vi "HEWH RLT PRAT.vi"() -> ()   [LabVIEW 2023] (continued)
      n65 = call "HEWH GEA Notifier.vi"("Status"=UTILITY_Notifier."Set", "error in (no error)"=w173, "name (unnamed)"="GEA_B") -> ("error out"=w172:errorcluster)  [unwired: 7 in, 1 out]
      n66 = call "HEWH GEA Notifier.vi"("Status"=UTILITY_Notifier."Set", "error in (no error)"=w172, "name (unnamed)"="GEA_C") -> ("error out"=w171:errorcluster)  [unwired: 7 in, 1 out]
      n67 = call "HEWH GEA Notifier.vi"("Status"=UTILITY_Notifier."Set", "error in (no error)"=w171, "name (unnamed)"="GEA_D") -> ("error out"=w141:errorcluster)  [unwired: 7 in, 1 out]
      n68 = Bundle By Name(cluster="File Locations In", "General Setup Paths.Tool Base Path"=w188) -> (w191:T3)
      n69 = call "UTILITY String Notifier.vi"("Status"=UTILITY_Notifier."Set", "error in (no error)"=w141, "Set Status"="", "name (unnamed)"="GasThermalEff") -> ("error out"=w140:errorcluster)  [unwired: 6 in, 1 out]
      n70 = call "HEWH Gas Notifier.vi"("Status"=UTILITY_Notifier."Set", "error in (no error)"=w140, "name (unnamed)"="GasData") -> ("error out"=w134:errorcluster)  [unwired: 7 in, 1 out]
      n71 = case shown="\"Four Stations\"" w187 {
        tunnel: [w251 w265] -> w185
        tunnel: [w251 w264] -> w184
        tunnel: [w251 w263] -> w183
        tunnel: [w249 w262] -> w108
        tunnel: [w249 w261] -> w107
        tunnel: [w249 w260] -> w106
        tunnel: w191 -> [_ w256]
        tunnel: [w250 w259] -> w167
        tunnel: [w250 w258] -> w166
        tunnel: [w250 w257] -> w165
        tunnel: errorcluster {"status"=FALSE, "code"=0, "source"=""} ("error out") -> [w248 w252]
        tunnel: [w248 w253] -> w129
        frame "Single Station", Default {
          w249 = refnum<k24> refnum (".NET Refnum in")
          w250 = T3 {"General Setup Paths"={"Calibration File Path"=path "", "DOE Capacity Path"=path "", "Data Folder Path"=path "", "RLT Backup Data Path"=path "", "Tool Base Path"=path "", "General Startup Config Path"=path "", "File Save Previous Run Path"=path "", "File Save Configuration Data Path"=path ""}, "Data File Paths"={"Data File Path"=path "", "Debug File Path"=path "", "Bus Log Path"=path "", "Current"=path "", "Summary"=path ""}, "New Summary Created"=FALSE, "Check Location Interval (Second)"=0} ("File Locations Out")
          w251 = T31 {"Appliance Details"={"FileVersionInfo"={"FileVersion"="", "ProductName"="", "InternalName"="", "CompanyName"="", "LegalCopyright"="", "FileDescription"=""}, "Dishwasher Info"={"Open Cup Weight (gm):"=0.0, "Auto Cup Weight (gm):"=0.0, "Detergent-Dish:"="", "Inlet Temperature-Dish:"="", "Cycle Mode-Dish:"="", "Unit Control-Dish:"="", "Manufacturer-Dish:"=""}, "Washer Info"={"Hot Water Temperature (Fahrenheit):"="", "Cold Water Temperature (Fahrenheit):"="", "Capacity (cu.ft):"=0.0, "Initial Cloth Weight:"=0.0, "Cloth Lot:"=0, "Model Family:"="", "Program Name:"="", "Cycle Selection:"="", "Wash Temperature:"="", "Rinse Temperature:"="", "Load Size:"=""}, "File Name Output Array"=[], "Calibration Output Array"=[], "Appliance Common"={"Engineer:"="", "Model Number:"="", "Serial Number:"="", "Comments:"="", "Station ID:"="", "Technician:"="", "TR Number:"="", "Lab ID:"="", "Voltage:"="", "Water Pressure (PSI):"="", "Test Date:"="", "Computer Name:"="", "IP Address:"="", "Ambient RH:"="", "Frequency:"="", "Build:"="", "Filename:"="", "Test Type:"="", "Load Run #:"=0, "Ambient Temperature (F):"="", "File Path:"=path "", "Cycles Per Year"=60}, "Water Heater"={"Heating Mode:"=""}, "Dryer"={"Heat Setting:"="", "Washer Water Temperature (60 ± 5°F):"=60, "Water Hardness (PPM):"=17, "Dryness Setting:"="", "Dryer Type:"="", "Exhaust:"="", "Drying Cycle:"="", "Load Type:"="", "Nominal Load Weight"="", "Dryer Initial IMC Data"={"Measured IMC (lbs)"=7.0, "Actual Initial RMC (%)"=7.0, "RMC (Desired %)"=100.0, "Bone Dry Wt(lbs)"=7.0, "Tolerance(%)"=5.0, "Actual Final RMC (%)"=0.0, "CEF (lbf/kWh)"=0.0, "Minimum Weight (lbf)"=0.0, "Average Weight (lbf)"=0.0, "Maximum Weight (lbf)"=0.0, "Measured IMC In Range?"=FALSE, "Moisture Reduction Factor"=55.5, "Field Use Factor"=1.04, "Empty Dryer Cold Weigth"=0.0, "Energy Standard"=enum."D2-Automatic Dryer", "Weight Cloth (lbs)"=0.0, "Relative Moisture Content (%)"=0.0, "Relative Moisture Content - Avg (%)"=0.0}}}, "Display Data (RLT)"={"Status Color"=0, "Serial Number Display"="", "Cycle Count Display"=0, "Station Label Display"="", "Current Run Start Time Display"=0.0, "Board ID Display"="", "RPM Display"=0, "Current Display"=0.0, "Current Path Display"=path "", "Saving Display"=FALSE, "Unit Type Display"=enum."", "Total Time On Display"=0.0, "UI Button"=FALSE}} ("Main Washer Display Out")
          # "GEA Information Out"
        }
        frame "Four Stations" {
          n72 = call "UTILITY Read Config File Start BUS.vi"("Error In"=w252, "Station ID"="StationD", "File Locations In"=w256) -> ("Error Out"=w255:errorcluster, "Main Washer Display Out"=w263:T31, "GEA3 Reference Out"=w260:refnum<k24>, "File Locations Out"=w257:T3)  [unwired: 5 in]
          n73 = call "UTILITY Read Config File Start BUS.vi"("Error In"=w255, "Station ID"="StationC", "File Locations In"=w256) -> ("Error Out"=w254:errorcluster, "Main Washer Display Out"=w264:T31, "GEA3 Reference Out"=w261:refnum<k24>, "File Locations Out"=w258:T3)  [unwired: 5 in]
          n74 = call "UTILITY Read Config File Start BUS.vi"("Error In"=w254, "Station ID"="StationB", "File Locations In"=w256) -> ("Error Out"=w253:errorcluster, "Main Washer Display Out"=w265:T31, "GEA3 Reference Out"=w262:refnum<k24>, "File Locations Out"=w259:T3)  [unwired: 5 in]
        }
      }
      n75 = call "UTILITY Boolean Notifier.vi"("Status"=UTILITY_Notifier."Set", "error in (no error)"=w134, "Set Status"=FALSE, "name (unnamed)"="Splash") -> ("error out"=w121:errorcluster)  [unwired: 6 in, 1 out]
      n76 = call "HEWH MW100 Data.vi"("Status"=UTILITY_Notifier."Set", "error in (no error)"=w121, "name (unnamed)"="MW100") -> ("error out"=w120:errorcluster)  [unwired: 7 in, 1 out]
      n77 = call "HEWH Emerson Data.vi"("Status"=UTILITY_Notifier."Set", "error in (no error)"=w120, "name (unnamed)"="Emerson") -> ("error out"=w114:errorcluster)  [unwired: 7 in, 1 out]
      n78 = call "UTILITY String Notifier.vi"("Status"=UTILITY_Notifier."Set", "error in (no error)"=w114, "Set Status"="", "name (unnamed)"="Scan_Rate") -> ("error out"=w111:errorcluster)  [unwired: 6 in, 1 out]
      n79 = call "UTILITY Read Config File Start BUS.vi"("Error In"=w129, "Station ID"="StationA", "File Locations In"=w191) -> ("Main Washer Display Out"=w186:T31, "GEA3 Reference Out"=w109:refnum<k24>, "File Locations Out"=w168:T3)  [unwired: 5 in, 1 out]
      n80 = call "HEWH HHV Notifier.vi"("Status"=UTILITY_Notifier."Set", "error in (no error)"=w111, "name (unnamed)"="HHVData") -> ("error out"=w104:errorcluster)  [unwired: 7 in, 1 out]
      n81 = Obtain Notifier(name (unnamed)="SplashScreen", notification data type=FALSE ("Init Complete"), error in (no error)=w104) -> (notifier out=w130:refnum<notifier>, error out=w131:errorcluster)  [unwired: 1 in, 1 out]
    }
    frame Enabled {
    }
  }
  n82 = disable-structure shown="Disabled" {
    disable-tunnel: w100 -> [w289 _]
    disable-tunnel: w99 -> [w288 _]
    disable-tunnel: w96 -> [w286 _]
    disable-tunnel: w95 -> [w285 _]
    disable-tunnel: w57 -> [w284 _]
    frame Disabled {
      # "Do the stuff associated with a draw"
      n83 = while {
        tunnel: w284 -> [w290]
        tunnel: [w290] -> w287
        stop <- w291 stop-if-true
        # "Make sure you get correct info during start"
        n84 = local read "Start Draw Loop"() -> (w291:bool)
        n85 = Wait Until Next ms Multiple(millisecond multiple=u32 250) -> ()  [unwired: 1 out]
      }
      n86 = while {
        tunnel: w287 -> [w303]
        tunnel: [w312] -> _
        tunnel: w286 -> [w311]
        tunnel: w289 -> [w298]
        tunnel: w288 -> [w299]
        tunnel: w285 -> [w295]
        i -> [w310]
        stop <- w309 stop-if-true
        n87 = Dequeue Element(queue=w298, error in (no error)=w303) -> (element=w300:T81, error out=w302:errorcluster)  [unwired: 1 in, 2 out]
        n88 = local read "Finish"() -> (w309:bool)
        n89 = Unbundle By Name(w300) -> ("Start Draw"=w296:bool, "Station ID"=w301:T26, "Station Draw Info"=w297:T15, "Send Condition"=w294:T2, "Disable Purge Pressurization"=w293:bool)
        "Start Draw" <- w296
        n90 = Wait Until Next ms Multiple(millisecond multiple=u32 100) -> ()  [unwired: 1 out]
        n91 = case shown="\"A\", Default" w301 {
          tunnel: [w313 w314 w315 w316] -> w307
          frame "A", Default {
            n92 = local read "Disable Station 1"() -> (w313:T34)
          }
          frame "B" {
            n93 = local read "Disable Station 2"() -> (w314:T34)
          }
          frame "C" {
            n94 = local read "Disable Station 3"() -> (w315:T34)
          }
          frame "D" {
            n95 = local read "Disable Station 4"() -> (w316:T34)
          }
        }
        n96 = Equal?(x=HEWH_RLT_Station_Disable."Enable Station", y=w307) -> (x = y?=w305:bool)
        n97 = And(x=w296, y=w305) -> (x .and. y?=w304:bool)
        n98 = case shown="True" w304 {
          tunnel: w302 -> [w317 w347]
          tunnel: [w317 w321] -> w312
          tunnel: w311 -> [_ w343]
          tunnel: w301 -> [_ w339]
          tunnel: w299 -> [_ w323]
          tunnel: w297 -> [_ w335]
          tunnel: w295 -> [_ w324]
          tunnel: w294 -> [_ w338]
          tunnel: w293 -> [_ w334]
          frame False {
          }
          frame True {
            # "This is everything required to draw water"
            n99 = flat-sequence {
              tunnel: w347 -> [w457]
              tunnel: [w457] -> w333
              frame #0 {
                n100 = property on="Scan Rate (Seconds)" class="DigNum (strict)"("Value"=T11 30.0 ("Scan Rate (Seconds)")) -> ()  [unwired: 2 in, 2 out]
                n101 = local write "Draw Complete"(FALSE ("Draw Complete")) -> ()
              }
            }
            n102 = local read "Intellifaucet Open Greater 2.2 GPM"() -> (w326:dbl)
            n103 = local read "Intellifaucet Open Less  2.2 GPM"() -> (w327:dbl)
            n104 = local read "Intellifaucet Open Less 1_7 GPM"() -> (w328:dbl)
            n105 = local read "Intellifaucet Open Less 1 GPM"() -> (w329:dbl)
            n106 = local read "Ritter Gas Drum Meter"() -> (w318:bool)
            n107 = control-ref of="Scan Rate (Seconds)"() -> (w319:refnum<vi>)
            n108 = local read "K-Factor (Flow)"() -> (w337:dbl)
            n109 = local read "Test Fixture Hardware Draw Loop"() -> (w332:T55)
            n110 = local read "Intellifaucet Type"() -> (w336:string)
            n111 = local read "Pressurize Tank?"() -> (w341:bool)
            n112 = local read "K-Factor (Temperature)"() -> (w340:dbl)
            n113 = case shown="\"A\", Default" w339 {
              tunnel: w333 -> [w371 w394 w417 w440]
              tunnel: "Purge Time (Seconds)" -> [w370 w391 w414 w439]
              tunnel: [w361 w384 w407 w430] -> w346
              tunnel: w335 -> [w369 w390 w409 w438]
              tunnel: "Skip Purge" -> [w367 w392 w416 w437]
              tunnel: "Skip Draw" -> [w366 w393 w415 w436]
              tunnel: w343 -> [w368 w387 w412 w435]
              tunnel: w341 -> [w363 w386 w411 w432]
              tunnel: w340 -> [w362 w385 w410 w431]
              tunnel: w338 -> [w360 w383 w406 w429]
              tunnel: w337 -> [w359 w382 w405 w428]
              tunnel: w336 -> [w358 w381 w404 w427]
              tunnel: w334 -> [w357 w380 w403 w426]
              tunnel: w332 -> [w356 w379 w402 w425]
              tunnel: "Pressurization Time (sec)" -> [w355 w378 w401 w424]
              tunnel: "NOx Purge Time" -> [w354 w377 w400 w423]
              tunnel: w329 -> [w353 w376 w399 w422]
              tunnel: w328 -> [w352 w375 w398 w421]
              tunnel: w327 -> [w351 w374 w397 w420]
              tunnel: w326 -> [w350 w373 w396 w419]
              tunnel: w319 -> [w349 _ _ _]
              tunnel: w318 -> [w348 w372 w395 w418]
              frame "A", Default {
                n114 = local read "Core HEWH Data Input A"() -> (w365:T13)
                n115 = call "HEWH Purge Draw Sequence.vi"("Intellifaucet Open Less 1 GPM"=w353, "Purge Time (Seconds)"=w370, "Intellifaucet Open Less 1_7 GPM"=w352, "Station Draw Info"=w369, "Current Cond"=w360, "Intellifaucet Open Less  2.2 GPM"=w351, "Intellifaucet Open Greater 2.2 GPM"=w350, "Error In"=w371, "Skip Purge"=w367, "Core HEWH Data Input"=w365, "Scan Rate (Seconds)"=w349, "Disable Purge Pressurization"=w357, "Skip Draw"=w366, "MW100 Sema"=w368, "K-Factor (Intellifaucet)"=w362, "Pressurize Tank while Heating?"=w363, "Intellifaucet Type"=w358, "Ritter Gas Drum Meter"=w348, "Test Fixture Hardware"=w356, "NOx Purge Time"=w354, "K-Factor (Flow)"=w359, "Pressurization Time (sec)"=w355) -> ("Core HEWH Data out"=→"Station A Update":T13, "Error Out"=w361:errorcluster)  [unwired: 4 in]
              }
              frame "B" {
                n116 = local read "Core HEWH Data Input B"() -> (w389:T13)
                n117 = call "HEWH Purge Draw Sequence.vi"("Intellifaucet Open Less 1 GPM"=w376, "Purge Time (Seconds)"=w391, "Intellifaucet Open Less 1_7 GPM"=w375, "Station Draw Info"=w390, "Current Cond"=w383, "Intellifaucet Open Less  2.2 GPM"=w374, "Intellifaucet Open Greater 2.2 GPM"=w373, "Error In"=w394, "Skip Purge"=w392, "Core HEWH Data Input"=w389, "Disable Purge Pressurization"=w380, "Skip Draw"=w393, "MW100 Sema"=w387, "K-Factor (Intellifaucet)"=w385, "Pressurize Tank while Heating?"=w386, "Intellifaucet Type"=w381, "Ritter Gas Drum Meter"=w372, "Test Fixture Hardware"=w379, "NOx Purge Time"=w377, "K-Factor (Flow)"=w382, "Pressurization Time (sec)"=w378) -> ("Core HEWH Data out"=→"Station B Update":T13, "Error Out"=w384:errorcluster)  [unwired: 5 in]
              }
              frame "C" {
                n118 = local read "Core HEWH Data Input C"() -> (w408:T13)
                n119 = call "HEWH Purge Draw Sequence.vi"("Intellifaucet Open Less 1 GPM"=w399, "Purge Time (Seconds)"=w414, "Intellifaucet Open Less 1_7 GPM"=w398, "Station Draw Info"=w409, "Current Cond"=w406, "Intellifaucet Open Less  2.2 GPM"=w397, "Intellifaucet Open Greater 2.2 GPM"=w396, "Error In"=w417, "Skip Purge"=w416, "Core HEWH Data Input"=w408, "Disable Purge Pressurization"=w403, "Skip Draw"=w415, "MW100 Sema"=w412, "K-Factor (Intellifaucet)"=w410, "Pressurize Tank while Heating?"=w411, "Intellifaucet Type"=w404, "Ritter Gas Drum Meter"=w395, "Test Fixture Hardware"=w402, "NOx Purge Time"=w400, "K-Factor (Flow)"=w405, "Pressurization Time (sec)"=w401) -> ("Core HEWH Data out"=→"Station C Update":T13, "Error Out"=w407:errorcluster)  [unwired: 5 in]
              }
              frame "D" {
                n120 = local read "Core HEWH Data Input D"() -> (w434:T13)
                n121 = call "HEWH Purge Draw Sequence.vi"("Intellifaucet Open Less 1 GPM"=w422, "Purge Time (Seconds)"=w439, "Intellifaucet Open Less 1_7 GPM"=w421, "Station Draw Info"=w438, "Current Cond"=w429, "Intellifaucet Open Less  2.2 GPM"=w420, "Intellifaucet Open Greater 2.2 GPM"=w419, "Error In"=w440, "Skip Purge"=w437, "Core HEWH Data Input"=w434, "Disable Purge Pressurization"=w426, "Skip Draw"=w436, "MW100 Sema"=w435, "K-Factor (Intellifaucet)"=w431, "Pressurize Tank while Heating?"=w432, "Intellifaucet Type"=w427, "Ritter Gas Drum Meter"=w418, "Test Fixture Hardware"=w425, "NOx Purge Time"=w423, "K-Factor (Flow)"=w428, "Pressurization Time (sec)"=w424) -> ("Core HEWH Data out"=→"Station D Update":T13, "Error Out"=w430:errorcluster)  [unwired: 5 in]
              }
            }
            n122 = flat-sequence {
              tunnel: w346 -> [w444]
              tunnel: w324 -> [w443]
              tunnel: [w442] -> w322
              tunnel: [w449] -> w325
              tunnel: w323 -> [w448]
              tunnel: w322 -> [w447]
              tunnel: w325 -> [w451]
              tunnel: [w451] -> w320
              tunnel: [w454] -> w321
              tunnel: w320 -> [w454]
              frame #0 {
                # "Increment cycle"
                n123 = Generate User Event(priority (normal)=usereventprio."high priority", user event=w443, event data cluster=TRUE ("Draw Start"), error in=w444) -> (error out=w442:errorcluster)  [unwired: 1 out]
              }
              frame #1 {
                # "Update draw stats"
                n124 = Generate User Event(priority (normal)=usereventprio."normal priority", user event=w448, event data cluster=TRUE ("event data"), error in=w447) -> (error out=w449:errorcluster)  [unwired: 1 out]
              }
              frame #2 {
              }
              frame #3 {
                n125 = property on="Scan Rate (Seconds)" class="DigNum (strict)"("Value"="Scan Rate (Default)") -> ()  [unwired: 2 in, 2 out]
                "Draw Complete" <- TRUE ("Draw Complete")
              }
            }
          }
        }
        "Draw Loop" <- w310
      }
    }
    frame Enabled {
    }
  }
  n126 = flat-sequence {
    tunnel: w57 -> [w459]
    tunnel: [w459] -> w74
    frame #0 {
      n127 = while {
        stop <- TRUE stop-if-true
        n128 = disable-structure shown="Disabled" {
          frame Disabled {
            n129 = local read "DAQ Complete"() -> ()  [unwired: 1 out]
          }
          frame Enabled {
          }
        }
        n130 = Wait (ms)(milliseconds to wait=u32 250) -> ()  [unwired: 1 out]
      }
      n131 = local write "Enable Auto Control"(FALSE ("Enable Auto Control")) -> ()
    }
  }
  n132 = disable-structure shown="Disabled" {
    disable-tunnel: [w466 _] -> w81
    disable-tunnel: w57 -> [w462 _]
    frame Disabled {
      # "Display messages. I need to work on this. \n\nIt was lower priority."
      n133 = Obtain Queue(name (unnamed)="ScanRate", element data type=FALSE, error in (no error)=w462) -> (queue out=w466:refnum<queue>, error out=w465:errorcluster)  [unwired: 2 in, 1 out]
      n134 = while {
        tunnel: w466 -> [w475]
        tunnel: w465 -> [w474]
        tunnel: [w473] -> w464
        tunnel: [w472] -> w463
        i -> [w469]
        stop <- w476 stop-if-true
        n135 = local read "DAQ Finished"() -> (w476:bool)
        n136 = call "HEWH Scan Rate Loop Trigger.vi"("Scan Rate (Seconds)"="Scan Rate (Seconds)", "Loop Index Input"=w469) -> ("Loop Trigger"=w470:bool)  [unwired: 7 in, 2 out]
        n137 = Enqueue Element(queue=w475, element=w470, error in (no error)=w474) -> (queue out=w472:refnum<queue>, error out=w473:errorcluster)  [unwired: 1 in, 1 out]
      }
      n138 = while {
        i -> [w477]
        stop <- w496 stop-if-true
        w491 = UTILITY_Notifier."Read" ("Status")
        n139 = call "UTILITY String Notifier.vi"("Status"=w491, "name (unnamed)"="Message") -> ("error out"=w495:errorcluster, "latest notification"=w483:string)  [unwired: 8 in]
        "Message" <- w483
        n140 = local read "Disable Station 1"() -> (w481:T34)
        n141 = call "UTILITY String Notifier.vi"("Status"=w491, "error in (no error)"=w495, "name (unnamed)"="MessageA") -> ("error out"=w494:errorcluster, "latest notification"=w486:string)  [unwired: 7 in]
        n142 = case shown="\"Enable Station\"" w481 {
          tunnel: w486 -> [_ w514]
          tunnel: w483 -> [_ w512]
          frame "Disable Station (No Draw)", Default {
          }
          frame "Enable Station" {
            n143 = call "HEWH Message Filter.vi"("Main Display?"=TRUE, "Station Message"=w514, "Main Message"=w512) -> ("Combined Message"=→"Message A" →"Message A Detail":string)  [unwired: 7 in, 1 out]
          }
        }
        n144 = local read "Disable Station 2"() -> (w480:T34)
        n145 = call "UTILITY String Notifier.vi"("Status"=w491, "error in (no error)"=w494, "name (unnamed)"="MessageB") -> ("error out"=w493:errorcluster, "latest notification"=w485:string)  [unwired: 7 in]
        n146 = case shown="\"Disable Station (No Draw)\", Default" w480 {
          tunnel: w485 -> [_ w510]
          tunnel: w483 -> [_ w508]
          frame "Disable Station (No Draw)", Default {
          }
          frame "Enable Station" {
            n147 = call "HEWH Message Filter.vi"("Main Display?"=TRUE, "Station Message"=w510, "Main Message"=w508) -> ("Combined Message"=→"Message B" →"Message B Detail":string)  [unwired: 7 in, 1 out]
          }
        }
        n148 = local read "Disable Station 3"() -> (w479:T34)
        n149 = call "UTILITY String Notifier.vi"("Status"=w491, "error in (no error)"=w493, "name (unnamed)"="MessageC") -> ("error out"=w492:errorcluster, "latest notification"=w484:string)  [unwired: 7 in]
        n150 = case shown="\"Disable Station (No Draw)\", Default" w479 {
          tunnel: w484 -> [_ w506]
          tunnel: w483 -> [_ w504]
          frame "Disable Station (No Draw)", Default {
          }
          frame "Enable Station" {
            n151 = call "HEWH Message Filter.vi"("Main Display?"=TRUE, "Station Message"=w506, "Main Message"=w504) -> ("Combined Message"=→"Message C" →"Message C Detail":string)  [unwired: 7 in, 1 out]
          }
        }
        n152 = local read "Disable Station 4"() -> (w478:T34)
        n153 = call "UTILITY String Notifier.vi"("Status"=w491, "error in (no error)"=w492, "name (unnamed)"="MessageD") -> ("latest notification"=w482:string)  [unwired: 7 in, 1 out]
        n154 = case shown="\"Enable Station\"" w478 {
          tunnel: w483 -> [_ w502]
          tunnel: w482 -> [_ w501]
          frame "Disable Station (No Draw)", Default {
          }
          frame "Enable Station" {
            n155 = call "HEWH Message Filter.vi"("Main Display?"=TRUE, "Station Message"=w501, "Main Message"=w502) -> ("Combined Message"=→"Message D" →"Message D Detail":string)  [unwired: 7 in, 1 out]
          }
        }
        n156 = Wait Until Next ms Multiple(millisecond multiple=u32 1000) -> ()  [unwired: 1 out]
        n157 = local read "DAQ Finished"() -> (w496:bool)
        "GEA3 Read Message Loop" <- w477
      }
      n158 = Release Queue(queue=w463, error in (no error)=w464) -> ()  [unwired: 1 in, 3 out]
    }
    frame Enabled {
    }
  }
  n159 = disable-structure shown="Disabled" {
    disable-tunnel: w102 -> [w531 _]
    disable-tunnel: w98 -> [w529 _]
    disable-tunnel: w96 -> [w528 _]
    disable-tunnel: w94 -> [w527 _]
    disable-tunnel: w93 -> [w526 _]
    disable-tunnel: w92 -> [w525 _]
    disable-tunnel: w91 -> [w524 _]
    disable-tunnel: w90 -> [w523 _]
    disable-tunnel: w87 -> [w522 _]
    disable-tunnel: w86 -> [w521 _]
    disable-tunnel: w85 -> [w520 _]
    disable-tunnel: w84 -> [w519 _]
    disable-tunnel: w83 -> [w518 _]
    disable-tunnel: w82 -> [w517 _]
    disable-tunnel: w81 -> [w516 _]
    frame Disabled {
      # "Get data from system"
      n160 = while "Data Acquisition Steps" {
        shift-right: [w552] -> _
        shift-left: _ -> [w551]
        shift-right: [w555] -> w515
        shift-left: w518 -> [w550]
        shift-right: [w554] -> _
        shift-left: w531 -> [w556]
        tunnel: w528 -> [w549]
        tunnel: w529 -> [w548]
        shift-right: [w544] -> _
        shift-left: string[] [] -> [w547]
        tunnel: w527 -> [w543]
        tunnel: w526 -> [w542]
        tunnel: w525 -> [w541]
        tunnel: w524 -> [w540]
        tunnel: w523 -> [w539]
        tunnel: w522 -> [w538]
        tunnel: w521 -> [w537]
        tunnel: w520 -> [w536]
        tunnel: w519 -> [w535]
        tunnel: w517 -> [w534]
        tunnel: w516 -> [w533]
        i -> [w532]
        stop <- w553 stop-if-true
        # "Data Acquisition Steps"
        n161 = call <vilib>:"Parse State Queue__JKI_lib_State_Machine.vi"("State Queue"=w556, "Error In (no error)"=w550) -> ("Remaining States"=w558:string, "Current State"=w546:string, "Arguments"=w557:string)  [unwired: 11 in]
        "DAQ State" <- w546
        n162 = case shown="\"Get Gas Data\"" w546 {
          selector: w546 -> [_ w681 _ _ _ _ _ _ _ _ _ _ _ _ _ _ _ _ _ _ _ _ _ _ _ _ _ _ _ _ _ _ _ _ _ _ _ _ _ _ _ _ _ _ _ _ _]
          tunnel: w558 -> [w571 w684 w696 w704 w716 w745 w792 w814 w833 w840 w850 w887 w913 w929 w938 w942 w955 w1005 w1041 w1077 w1113 w1136 w1153 w1170 w1187 w1203 w1220 w1245 w1327 w1352 w1379 w1398 w1428 w1458 w1487 w1540 w1573 w1601 w1629 w1657 w1694 w1709 w1733 w1757 w1781 w1792 w1819]
          tunnel: w557 -> [_ _ _ _ _ _ _ _ _ _ _ _ _ _ _ _ _ _ _ _ _ _ _ _ _ _ _ _ _ _ _ _ _ _ _ _ _ _ _ _ _ _ _ _ _ _ _]
          tunnel: [w569 w686 errorcluster {"status"=FALSE, "code"=0, "source"=""} ("error out") w700 w714 w718 w784 w800 w825 w838 w848 w877 w910 w922 w930 w940 w943 w995 w1033 w1069 w1105 w1128 w1148 w1165 w1182 w1191 w1207 w1239 w1318 w1338 w1365 w1395 w1424 w1454 w1483 w1524 w1553 w1599 w1627 w1655 w1692 w1700 w1724 w1748 w1772 w1793 w1805] -> w555
          tunnel: w550 -> [w564 w685 w692 w701 w714 w718 w775 w798 w823 w838 w848 w885 w911 w923 w934 w940 w943 w997 w1035 w1071 w1107 _ w1140 w1157 w1176 w1191 w1206 w1243 w1308 w1338 w1366 w1396 w1425 w1455 w1484 w1533 w1553 w1599 w1627 w1655 w1692 w1696 w1720 w1744 w1769 w1793 w1817]
          tunnel: [w570 w683 w695 w703 w715 w744 w791 w813 w832 w839 w849 w886 w912 w928 w937 w941 w954 w1004 w1040 w1076 w1112 w1137 w1154 w1171 w1188 w1202 w1219 w1244 w1326 w1351 w1378 w1397 w1427 w1457 w1486 w1539 w1572 w1600 w1628 w1656 w1693 w1708 w1732 w1756 w1780 w1792 w1819] -> w554
          tunnel: [_ _ _ w698 _ _ _ _ _ _ _ _ _ _ _ _ _ _ _ _ _ _ _ _ _ _ _ _ _ _ _ _ _ _ _ _ _ _ _ _ _ _ _ _ _ _ _] -> w553
          tunnel: [w568 w680 w691 w702 w713 w729 w790 w812 w831 w837 w844 w880 w905 w927 w936 w939 w953 w1003 w1039 w1075 w1111 w1135 w1152 w1169 w1186 w1201 w1218 w1236 w1325 w1350 w1377 w1394 w1423 w1453 w1482 w1538 w1567 w1592 w1618 w1648 w1691 w1702 w1725 w1749 w1773 w1791 w1798] -> w552
          tunnel: w551 -> [w567 w680 w691 w702 w713 _ w781 w812 w831 w837 w845 w882 w905 w927 w936 w939 w950 w1000 w1038 w1074 w1110 w1129 w1151 w1168 w1185 w1196 w1213 w1238 w1304 w1345 w1372 w1392 w1426 w1456 w1485 w1538 w1568 w1593 w1619 w1649 w1690 w1703 w1726 w1750 w1774 w1791 w1799]
          tunnel: w549 -> [_ _ _ _ _ _ w771 w802 w827 _ _ _ _ _ w933 _ _ w996 w1034 w1070 w1106 _ _ _ _ _ _ _ _ _ _ _ _ _ _ _ _ _ _ _ _ _ _ _ _ _ _]
          tunnel: w548 -> [w566 _ _ _ _ _ _ _ _ _ _ _ _ _ _ _ _ _ _ _ _ _ _ _ _ _ _ _ _ _ _ _ _ _ _ _ _ _ _ _ _ _ _ _ _ _ _]
          tunnel: w543 -> [_ _ _ _ _ _ _ _ _ _ _ _ _ _ _ _ w949 _ _ _ _ _ _ _ _ _ _ _ _ _ _ _ _ _ _ _ _ _ _ _ _ _ _ _ _ _ _]
          tunnel: w542 -> [_ _ _ _ _ _ _ _ _ _ _ _ _ _ _ _ _ _ _ _ _ _ _ _ _ _ _ _ _ _ _ w1391 _ _ _ _ _ _ _ _ _ _ _ _ _ _ _]
          tunnel: w541 -> [_ _ _ _ _ _ _ _ _ _ _ _ _ _ _ _ _ _ _ _ _ _ _ _ _ _ _ _ _ _ _ _ w1421 _ _ _ _ _ _ _ _ _ _ _ _ _ _]
          tunnel: w540 -> [_ _ _ _ _ _ _ _ _ _ _ _ _ _ _ _ _ _ _ _ _ _ _ _ _ _ _ _ _ _ _ _ _ w1451 _ _ _ _ _ _ _ _ _ _ _ _ _]
          tunnel: w539 -> [_ _ _ _ _ _ _ _ _ _ _ _ _ _ _ _ _ _ _ _ _ _ _ _ _ _ _ _ _ _ _ _ _ _ w1480 _ _ _ _ _ _ _ _ _ _ _ _]
          tunnel: w538 -> [_ _ _ _ _ _ _ _ _ _ w843 _ _ _ _ _ _ _ _ _ _ _ _ _ _ _ _ _ _ _ _ _ _ _ _ _ _ _ _ _ _ _ _ _ _ _ _]
          tunnel: w537 -> [_ _ _ _ _ _ _ _ _ _ w847 _ _ _ _ _ _ _ _ _ _ _ _ _ _ _ _ _ _ _ _ _ _ _ _ _ _ _ _ _ _ _ _ _ _ _ _]
          tunnel: w536 -> [_ _ _ _ _ _ _ _ _ _ w842 _ _ _ _ _ _ _ _ _ _ _ _ _ _ _ _ _ _ _ _ _ _ _ _ _ _ _ _ _ _ _ _ _ _ _ _]
          tunnel: w535 -> [_ _ _ _ _ _ _ _ _ _ w841 _ _ _ _ _ _ _ _ _ _ _ _ _ _ _ _ _ _ _ _ _ _ _ _ _ _ _ _ _ _ _ _ _ _ _ _]
          tunnel: w534 -> [_ _ _ _ _ _ w777 _ _ _ _ _ _ _ _ _ _ _ _ _ _ _ _ _ _ _ _ _ _ _ _ _ _ _ _ _ _ _ _ _ _ _ _ _ _ _ _]
          tunnel: w533 -> [w563 _ _ _ _ _ _ _ _ _ _ _ _ _ _ _ _ _ _ _ _ _ _ _ _ _ _ _ _ _ _ _ _ _ _ _ _ _ _ _ _ _ _ _ _ _ _]
          frame "", "Idle" {
            n163 = event shown="[0] Timeout" {
              selector: w566 -> [_ _ _ _]
              dyn-events: _ -> [_ _ _ _]
              timeout: "DAQ Timeout" -> [_ _ _ _]
              tunnel: w571 -> [w584 w599 w613 w614]
              tunnel: [w574 w600 w613 w615] -> w570
              tunnel: w567 -> [w582 w601 w607 w617]
              tunnel: [w578 w597 w612 w618] -> w569
              tunnel: w564 -> [w577 w597 w612 w619]
              tunnel: [w582 w601 w606 w622] -> w568
              tunnel: w563 -> [w576 _ _ _]
              event Timeout {
                # "Trigger data save"
                n164 = event-data() -> ()  [unwired: 1 in, 1 out]
                n165 = Unbundle By Name(w582) -> ("Core HEWH Data Input A.LV Program"=w581:T25)
                n166 = Dequeue Element(queue=w576, error in (no error)=w577) -> (element=w579:bool, error out=w578:errorcluster)  [unwired: 1 in, 2 out]
                n167 = case shown="True" w579 {
                  tunnel: ["" w596] -> w573
                  tunnel: w581 -> [_ w595]
                  frame False {
                  }
                  frame True {
                    n168 = local read "Final Headers B"() -> (w588:bool)
                    n169 = local read "Log Data Output (D)"() -> (w591:bool)
                    n170 = local read "Final Headers A"() -> (w589:bool)
                    n171 = local read "Final Headers C"() -> (w587:bool)
                    n172 = local read "Final Headers D"() -> (w586:bool)
                    n173 = local read "Log Data Output (C)"() -> (w592:bool)
                    n174 = local read "Log Data Output (A)"() -> (w594:bool)
                    n175 = local read "Log Data Output (B)"() -> (w593:bool)
                    n176 = call "HEWH Create Save Data States.vi"("LV Program"=w595, "Data Loop?"=TRUE, "Final Headers A"=w589, "Final Headers C"=w587, "Log Data Output (C)"=w592, "Log Data Output (A)"=w594, "Log Data Output (D)"=w591, "Log Data Output (B)"=w593, "Final Headers B"=w588, "Final Headers D"=w586) -> ("SM States"=w596:string)  [unwired: 8 in, 1 out]
                  }
                }
                n177 = call "HEWH Build States.vi"("LV Program"=w581) -> ("SM States"=w583:string, "Get Gas Data"=w580:bool, "Vesta Connect"=w572:bool)  [unwired: 12 in]
                n178 = call <vilib>:"Add State(s) to Queue__jki_lib_state_machine.vi"("State(s) in Front (\"\")"=w583, "State(s) in (\"\")"=w584) -> ("States Out"=w575:string)  [unwired: 13 in]
                n179 = call <vilib>:"Add State(s) to Queue__jki_lib_state_machine.vi"("State(s) in Front (\"\")"=w573, "State(s) in (\"\")"=w575) -> ("States Out"=w574:string)  [unwired: 13 in]
              }
              event "Finish": Value Change {
                n180 = event-data() -> ()  [unwired: 1 in, 6 out]
                n181 = call <vilib>:"Add State(s) to Queue__jki_lib_state_machine.vi"("State(s) in Front (\"\")"="Shutdown Equipment\nExit", "State(s) in (\"\")"=w599) -> ("States Out"=w600:string)  [unwired: 13 in]
              }
              event User Event {
                n182 = event-data() -> ()  [unwired: 1 in, 5 out]
                n183 = local read "Station A Update"() -> (w608:T13)
                n184 = local read "Station B Update"() -> (w609:T13)
                n185 = local read "Station C Update"() -> (w610:T13)
                n186 = local read "Station D Update"() -> (w611:T13)
                n187 = Unbundle By Name(w608) -> ("Calc and Calibration"=w605:T24)
                n188 = Unbundle By Name(w609) -> ("Calc and Calibration"=w604:T24)
                n189 = Unbundle By Name(w610) -> ("Calc and Calibration"=w603:T24)
                n190 = Unbundle By Name(w611) -> ("Calc and Calibration"=w602:T24)
                n191 = Bundle By Name(cluster=w607, "Core HEWH Data Input A.Calc and Calibration"=w605, "Core HEWH Data Input B.Calc and Calibration"=w604, "Core HEWH Data Input C.Calc and Calibration"=w603, "Core HEWH Data Input D.Calc and Calibration"=w602) -> (w606:T88)
              }
              event User Event {
                n192 = event-data() -> ()  [unwired: 1 in, 5 out]
                n193 = local read "Station ID to Reset"() -> (w623:T26)
                n194 = case shown="\"A\", Default" w623 {
                  tunnel: w617 -> [w637 w651 w665 w679]
                  tunnel: [w636 w650 w664 w678] -> w622
                  tunnel: [w634 w642 w656 w669] -> w620
                  tunnel: w619 -> [w633 w644 w663 w677]
                  tunnel: [w632 w643 w662 w676] -> w618
                  tunnel: w617 -> [w630 w649 w660 w675]
                  frame "A", Default {
                    n195 = Unbundle By Name(w630) -> ("Core HEWH Data Input A.Calc and Calibration"=w628:T24)
                    n196 = local read "Log Data Output (A)"() -> (w635:bool)
                    n197 = local read "Updated File Path A"() -> (w631:T3)
                    n198 = local read "Reset Cycle Count"() -> (w626:bool)
                    n199 = call "HEWH Final Data Check.vi"("Station Message"="MessageA", "Input State"="Add Final Data A", "Calc and Calibration in"=w628, "error in (no error)"=w633, "Reset Cycle Count"=w626, "Updated File Path A in"=w631, "Log Data Output (A)"=w635) -> ("error out"=w632:errorcluster, "Updated File Path A out"=w629:T3, "Calc and Calibration out"=w627:T24, "Output State"=w634:string)  [unwired: 1 in]
                    n200 = Bundle By Name(cluster=w637, "Core HEWH Data Input A.Calc and Calibration"=w627, "File Locations A"=w629) -> (w636:T88)
                  }
                  frame "B" {
                    n201 = local read "Updated File Path B"() -> (w646:T3)
                    n202 = Unbundle By Name(w649) -> ("Core HEWH Data Input B.Calc and Calibration"=w648:T24)
                    n203 = local read "Log Data Output (B)"() -> (w647:bool)
                    n204 = local read "Reset Cycle Count"() -> (w645:bool)
                    n205 = call "HEWH Final Data Check.vi"("Station Message"="MessageB", "Input State"="Add Final Data B" ("State(s) in Front (\"\")"), "Calc and Calibration in"=w648, "error in (no error)"=w644, "Reset Cycle Count"=w645, "Updated File Path A in"=w646, "Log Data Output (A)"=w647) -> ("error out"=w643:errorcluster, "Updated File Path A out"=w639:T3, "Calc and Calibration out"=w640:T24, "Output State"=w642:string)  [unwired: 1 in]
                    n206 = Bundle By Name(cluster=w651, "Core HEWH Data Input B.Calc and Calibration"=w640, "File Locations B"=w639) -> (w650:T88)
                  }
                  frame "C" {
                    n207 = Unbundle By Name(w660) -> ("Core HEWH Data Input C.Calc and Calibration"=w659:T24)
                    n208 = local read "Updated File Path C"() -> (w658:T3)
                    n209 = local read "Log Data Output (C)"() -> (w661:bool)
                    n210 = local read "Reset Cycle Count"() -> (w655:bool)
                    n211 = call "HEWH Final Data Check.vi"("Station Message"="MessageC", "Input State"="Add Final Data C" ("State(s) in Front (\"\")"), "Calc and Calibration in"=w659, "error in (no error)"=w663, "Reset Cycle Count"=w655, "Updated File Path A in"=w658, "Log Data Output (A)"=w661) -> ("error out"=w662:errorcluster, "Updated File Path A out"=w653:T3, "Calc and Calibration out"=w654:T24, "Output State"=w656:string)  [unwired: 1 in]
                    n212 = Bundle By Name(cluster=w665, "Core HEWH Data Input C.Calc and Calibration"=w654, "File Locations C"=w653) -> (w664:T88)
                  }
                  frame "D" {
                    n213 = Unbundle By Name(w675) -> ("Core HEWH Data Input D.Calc and Calibration"=w674:T24)
                    n214 = local read "Log Data Output (D)"() -> (w673:bool)
                    n215 = local read "Updated File Path D"() -> (w672:T3)
                    n216 = local read "Reset Cycle Count"() -> (w671:bool)
                    n217 = call "HEWH Final Data Check.vi"("Station Message"="MessageD", "Input State"="Add Final Data D" ("State(s) in Front (\"\")"), "Calc and Calibration in"=w674, "error in (no error)"=w677, "Reset Cycle Count"=w671, "Updated File Path A in"=w672, "Log Data Output (A)"=w673) -> ("error out"=w676:errorcluster, "Updated File Path A out"=w667:T3, "Calc and Calibration out"=w668:T24, "Output State"=w669:string)  [unwired: 1 in]
                    n218 = Bundle By Name(cluster=w679, "Core HEWH Data Input D.Calc and Calibration"=w668, "File Locations D"=w667) -> (w678:T88)
                  }
                }
                n219 = call <vilib>:"Add State(s) to Queue__jki_lib_state_machine.vi"("State(s) in Front (\"\")"=w620, "State(s) in (\"\")"=w614) -> ("States Out"=w616:string)  [unwired: 13 in]
                n220 = call <vilib>:"Add State(s) to Queue__jki_lib_state_machine.vi"("State(s) in Front (\"\")"="Data: Update RLT Channels" ("State(s) in Front (\"\")"), "State(s) in (\"\")"=w616) -> ("States Out"=w615:string)  [unwired: 13 in]
              }
            }
          }
          frame Default {
            w689 = 42 items=["No error", "Argument error", "Memory is full", "Out of zone", "End of file", "File already open", "Generic file I/O error", "File not found", "File permission error", "Disk is full", "Duplicate path", "Too many files open", "System feature not enabled", "Resource file not found", "Cannot add resource", "Resource not found", "Image not found", "Image memory error", "Pen does not exist", "Config type invalid", "Config token not found", "Config parse error", "Config memory error", "Bad external code format", "Bad external code offset", "External code not present", "Null window", "Destroy window error", "Null menu", "Print aborted", "Bad print record", "Print driver error", "Windows error during printing", "Memory error during printing", "Print dialog error", "Generic print error", "Invalid device refnum", "Device not found", "Device parameter error", "Device unit error", "Cannot open device", "Device call aborted", "Generic error", "Cancelled by user", "Object ID too low", "Object ID too high", "Object not in heap", "Unknown heap", "Unknown object (invalid DefProc)", "Unknown object (DefProc not in table)", "Message out of range", "Invalid (null) method", "Unknown message", "Manager call not supported", "Bad address", "Network operation in progress", "Network operation timed out", "Connection is busy", "Network attribute not supported", "Network error", "Address in use", "System out of memory", "Connection aborted", "Connection refused", "Not connected", "Already connected", "Connection closed", "Initialization error (interapplication manager)", "Bad occurrence", "Wait on unbound occurrence handler", "Occurrence queue overflow", "Datalog type conflict", "Unused", "Unrecognized type (interapplication manager)", "Memory corrupt", "Failed to make temporary DLL", "Old CIN version", "Drag socket not found", "Failed to load drop-object", "Failed to register OLE object", "Failed to release OLE object", "Format specifier type mismatch", "Unknown format specifier", "Too few format specifiers", "Too many format specifiers", "Scan failed", "Newer CIN version", "Error converting to variant", "Runtime menu error", "Password tampered", "Variant attribute not found", "Incompatible variant data type", "Event data is not available", "Event Store is not present", "Occurrence is not found", "Event Queue is not created", "Event info is not available", "Refnum passed is NULL", "Error retrieving Class GUID", "Error retrieving CoClass GUID", "Error retrieving TypeLib GUID.", "Bad built application magic bytes.", "Specific driver is different from the specific driver associated with the Logical Name.", "There is no session opened to the class driver.", "Max Error", "MAX - Error with config objects", "MAX - Error loading configuration", "MAX - Group not supported"]
            # "Current State"
            # "Handle mistyped state name (developer tool)"
            n221 = Format Into String(format string="Software Exception: Unhandled State \"%s\"." ("message"), error in=w685, w681) -> (resulting string=w688:string, error out=w687:errorcluster)  [unwired: 1 in]
            n222 = call <vilib>:"Error Cluster From Error Code.vi"("show call chain? (False)"=TRUE, "error in (no error)"=w687, "error message (\"\")"=w688, "error code (0)"=w689) -> ("error out"=w686:errorcluster)  [unwired: 5 in]
            n223 = call <vilib>:"Add State(s) to Queue__jki_lib_state_machine.vi"("State(s) in (\"\")"=w684) -> ("States Out"=w683:string)  [unwired: 14 in]
          }
          frame "Error Handler" {
            # "Unhandled Error -- Display it"
            # "Clear error"
            n224 = call <vilib>:"General Error Handler.vi"("error in (no error)"=w692) -> ()  [unwired: 10 in, 5 out]
            n225 = call <vilib>:"Add State(s) to Queue__jki_lib_state_machine.vi"("State(s) in Front (\"\")"="/* Post Error States", "State(s) in (\"\")"=w696) -> ("States Out"=w695:string)  [unwired: 13 in]
          }
          frame "Exit" {
            n226 = flat-sequence {
              tunnel: w701 -> [w706]
              tunnel: [w706] -> w697
              tunnel: [w709] -> w699
              tunnel: w697 -> [w710]
              tunnel: [w712] -> w700
              tunnel: w699 -> [w712]
              tunnel: [TRUE] -> w698
              frame #0 {
                n227 = local read "Start Draw"() -> (w705:bool)
                n228 = case shown="True" w705 {
                  frame False {
                  }
                  frame True {
                    n229 = while {
                      stop <- w708 stop-if-true
                      n230 = local read "Draw Complete"() -> (w708:bool)
                      n231 = Wait Until Next ms Multiple(millisecond multiple=u32 100) -> ()  [unwired: 1 out]
                    }
                  }
                }
              }
              frame #1 {
                n232 = call "HEWH RLT Release Notifier References.vi"("error in (no error)"=w710) -> ("error out"=w709:errorcluster)  [unwired: 10 in]
              }
              frame #2 {
              }
            }
            n233 = call <vilib>:"Add State(s) to Queue__jki_lib_state_machine.vi"("State(s) in (\"\")"=w704) -> ("States Out"=w703:string)  [unwired: 14 in]
            "DAQ Finished" <- w698
          }
          frame "---------- Setup ----------" {
            n234 = call <vilib>:"Add State(s) to Queue__jki_lib_state_machine.vi"("State(s) in (\"\")"=w716) -> ("States Out"=w715:string)  [unwired: 14 in]
          }
          frame "Data: Initialize" {
            n235 = while {
              tunnel: ["Test Fixture Hardware"] -> w727
              tunnel: [w768] -> w743
              tunnel: [w767] -> w742
              tunnel: [w766] -> w741
              tunnel: [w765] -> w740
              tunnel: [w764] -> w739
              tunnel: [w763] -> w738
              tunnel: ["Core HEWH Data Input A"] -> w730
              tunnel: ["Core HEWH Data Input B"] -> w737
              tunnel: ["Core HEWH Data Input C"] -> w736
              tunnel: ["Core HEWH Data Input D"] -> w735
              tunnel: ["File Locations A"] -> w734
              tunnel: ["File Locations B"] -> w733
              tunnel: ["File Locations C"] -> w732
              tunnel: ["File Locations D"] -> w731
              tunnel: [w752] -> w725
              tunnel: [w751] -> w724
              tunnel: [w750] -> w723
              tunnel: [w749] -> w722
              tunnel: [w748] -> w721
              tunnel: [w747] -> w720
              tunnel: [w746] -> w717
              stop <- w762 stop-if-true
              w748 = dbl[][] []  # Plot Array C
              w747 = dbl[][] []  # Plot Array D
              w749 = dbl[][] []  # Plot Array B
              w750 = dbl[][] []  # Plot Array A
              w764 = string[][] []  # D Data Array
              w765 = string[][] []  # C Data Array
              w766 = string[][] []  # B Data Array
              w767 = string[][] []  # A Data Array
              w768 = string[][] []  # Save Data
              n236 = local read "Init Complete"() -> (w762:bool)
              n237 = Wait Until Next ms Multiple(millisecond multiple=u32 100) -> ()  [unwired: 1 out]
              n238 = local read "Analog Channel-List"() -> (w746:string)
              n239 = local read "RLT Station Channels"() -> (w763:T54)
              n240 = local read "Power Analyzer"() -> (w751:T12)
              n241 = local read "LV Program"() -> (w752:T25)
            }
            n242 = Bundle("Test Fixture Hardware"=w727, "Save Data"=w743, "A Data Array"=w742, "B Data Array"=w741, "C Data Array"=w740, "D Data Array"=w739, "RLT Station Channels"=w738, "Core HEWH Data Input A"=w730, "Core HEWH Data Input B"=w737, "Core HEWH Data Input C"=w736, "Core HEWH Data Input D"=w735, "File Locations A"=w734, "File Locations B"=w733, "File Locations C"=w732, "File Locations D"=w731, "Plot Array A"=w723, "Plot Array B"=w722, "Plot Array C"=w721, "Plot Array D"=w720) -> (w728:T88)  [unwired: 1 in]
            n243 = Unbundle By Name(w727) -> ("Analog Data.Yokogawa.MW100"=→"MW100":refnum<visa-resource-name>, "Power.Yokogawa.WT210.Power VISA Yokogawa WT210"=→"Yokogawa WT210":refnum<visa-resource-name>)
            n244 = Bundle By Name(cluster=w728, "Core HEWH Data Input A.HEWH Specific DAQ.Power Analyzer"=w724, "Core HEWH Data Input B.HEWH Specific DAQ.Power Analyzer"=w724, "Core HEWH Data Input C.HEWH Specific DAQ.Power Analyzer"=w724, "Core HEWH Data Input D.HEWH Specific DAQ.Power Analyzer"=w724, "Core HEWH Data Input A.LV Program"=w725, "Core HEWH Data Input B.LV Program"=w725, "Core HEWH Data Input C.LV Program"=w725, "Core HEWH Data Input D.LV Program"=w725, "Test Fixture Hardware.Analog Data.Agilent.TC Channels-List"=w717) -> (w729:T88)
            n245 = call <vilib>:"Add State(s) to Queue__jki_lib_state_machine.vi"("State(s) in (\"\")"=w745) -> ("States Out"=w744:string)  [unwired: 14 in]
          }
          frame "Initialize Equipment" {
            w785 = 0 ("Core HEWH Data Input A.Draw Count")
            # "Trigger Splash\nScreen"
            n246 = flat-sequence {
              tunnel: w775 -> [w795]
              tunnel: [w794] -> w778
              tunnel: w777 -> [w793]
              frame #0 {
                n247 = Send Notification(notification=TRUE, notifier=w793, error in (no error)=w795) -> (error out=w794:errorcluster)  [unwired: 1 out]
              }
            }
            n248 = Unbundle By Name(w781) -> ("Test Fixture Hardware"=w780:T55, "Core HEWH Data Input A"=w774:T13)
            n249 = local read "Station"() -> ()  [unwired: 1 out]
            n250 = call "HEWH Initialize Equipmet.vi"("Test Fixture Hardware"=w780, "Core HEWH Data"=w774, "Error In"=w778, "Pressurize Tank"="Pressurize Tank?", "Debug"=FALSE, "Refnum in"=w771) -> ("Test Fixture Hardware Out"=w770:T55, "Core HEWH Data Output"=w772:T13, "Error Out"=w779:errorcluster)  [unwired: 11 in]
            n251 = Unbundle By Name(w772) -> ("Module 4 Relay Status.MAIN POWER RELAY (CH 047)"=w776:bool)
            n252 = Bundle By Name(cluster=w781, "Core HEWH Data Input A.Station ID"=Station_ID_Selector."A", "Core HEWH Data Input B.Station ID"=Station_ID_Selector."B", "Core HEWH Data Input C.Station ID"=Station_ID_Selector."C", "Core HEWH Data Input D.Station ID"=Station_ID_Selector."D", "Core HEWH Data Input A.Draw Count"=w785, "Core HEWH Data Input B.Draw Count"=w785, "Core HEWH Data Input C.Draw Count"=w785, "Core HEWH Data Input D.Draw Count"=w785, "Test Fixture Hardware"=w770, "Core HEWH Data Input A"=w772) -> (w790:T88)
            n253 = call <vilib>:"Add State(s) to Queue__jki_lib_state_machine.vi"("State(s) in (\"\")"=w792) -> ("States Out"=w791:string)  [unwired: 14 in]
            n254 = local write "Main Power"(w776) -> ()
            n255 = call <vilib>:"Clear Errors.vi"("error in (no error)"=w779, "specific error code to clear (0: all)"=0) -> ("error out"=w784:errorcluster)  [unwired: 4 in, 1 out]
          }
          frame "UI Initialize" {
            n256 = Unbundle By Name(w812) -> ("Core HEWH Data Input A.Module 4 Relay Status.INLET VALVE RELAY (CH 050)"=w811:bool, "Core HEWH Data Input A.Module 4 Relay Status.PURGE VALVE RELAY (CH 048)"=w809:bool, "Core HEWH Data Input A.Module 4 Relay Status.OUTLET VALVE RELAY (CH 049)"=w808:bool, "Test Fixture Hardware"=w801:T55)
            n257 = case shown="False" w811 {
              tunnel: [T40 "ON" ("Inlet Valve A") T40 "OFF" ("Inlet Valve A")] -> w810
              frame False {
              }
              frame True {
              }
            }
            n258 = case shown="False" w809 {
              tunnel: [T41 "OFF" ("Drain Valve A") T41 "ON" ("Drain Valve A")] -> w806
              frame False {
              }
              frame True {
              }
            }
            n259 = case shown="False" w808 {
              tunnel: [T40 "ON" ("Inlet Valve A") T40 "OFF" ("Inlet Valve A")] -> w807
              frame False {
              }
              frame True {
              }
            }
            n260 = call "INTELLIFAUCET Driver.vi"("Test Fixture Hardware"=w801, "Mode"=INTELLIFAUCET_Set_Mode."Temp/Flow Relay", "Use General Conversion"=TRUE, "TEMP,FLOW"=INTELLIFAUCT_Temp_Flow."TEMP", "Flow Rate (GPM)"=0.0, "Error In"=w798, "Refnum in"=w802) -> ("Error Out"=w800:errorcluster)  [unwired: 6 in, 2 out]
            n261 = local write "Inlet Valve A"(w810) -> ()
            n262 = local write "Drain Valve A"(w806) -> ()
            n263 = local write "Outlet Valve A"(w807) -> ()
            n264 = local read "Manual HHV"() -> (w797:bool)
            n265 = case shown="False" w797 {
              frame False {
                w815 = T87."Disabled and Grayed Out" ("Disabled")
                n266 = property on="HHV-NG-Manual" class="DigNum (strict)"("DisabledEnum"=w815) -> ()  [unwired: 2 in, 2 out]
                n267 = property on="HHV-LP-Manual" class="DigNum (strict)"("DisabledEnum"=w815) -> ()  [unwired: 2 in, 2 out]
              }
              frame True {
                w816 = T87."Enabled" ("Disabled")
                n268 = property on="HHV-NG-Manual" class="DigNum (strict)"("DisabledEnum"=w816) -> ()  [unwired: 2 in, 2 out]
                n269 = property on="HHV-LP-Manual" class="DigNum (strict)"("DisabledEnum"=w816) -> ()  [unwired: 2 in, 2 out]
              }
            }
            n270 = call <vilib>:"Add State(s) to Queue__jki_lib_state_machine.vi"("State(s) in (\"\")"=w814) -> ("States Out"=w813:string)  [unwired: 14 in]
          }
          frame "UI Initialize 2" {
            n271 = Unbundle By Name(w831) -> ("Test Fixture Hardware"=w826:T55)
            n272 = call "INTELLIFAUCET Driver.vi"("Test Fixture Hardware"=w826, "Mode"=INTELLIFAUCET_Set_Mode."Temp/Flow Relay", "Use General Conversion"=TRUE, "TEMP,FLOW"=INTELLIFAUCT_Temp_Flow."FLOW", "Flow Rate (GPM)"=0.0, "Error In"=w823, "Refnum in"=w827) -> ("Error Out"=w825:errorcluster)  [unwired: 6 in, 2 out]
            n273 = call <vilib>:"Add State(s) to Queue__jki_lib_state_machine.vi"("State(s) in (\"\")"=w833) -> ("States Out"=w832:string)  [unwired: 14 in]
          }
          frame "UI Initialize 3" {
